vi "Convert Time to H_M_S.vi"(7 "Initial Scan Location":u32, 8 "error in":errorcluster, 10 "Tot. Timer Format":u16, 11 "Time Data String":string="Time Data String") -> (0 "error out":errorcluster, 1 "[sec]":dbl, 2 "[min]":dbl, 3 "[hr]":dbl, 5 "Offset Past Scan":u32)   [LabVIEW 2023]
doc: "Converts the Totalizer Timer data string into H:M:S doubles based on the time string format. A timer format of 2 is used if the Totalizer Timer is already outputting data in the H:M:S format.\n\nIf unsure of the format your Alicat uses, the output of the \"Read Measurement Format\" sub-VI will output the timer format for use with this sub-VI."
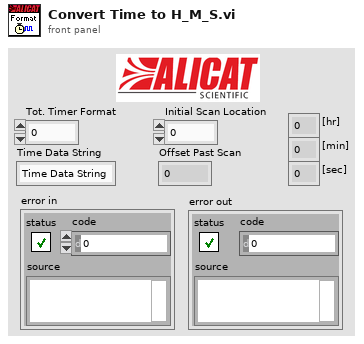
[diagram p1: front panel]
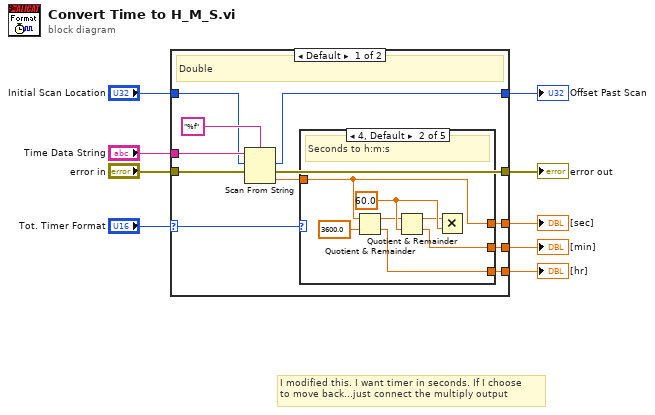
[diagram p0: block diagram]
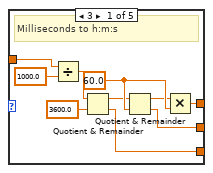
[diagram p2: hidden frame]
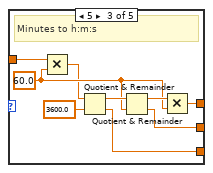
[diagram p3: hidden frame]
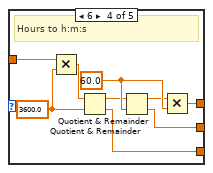
[diagram p4: hidden frame]
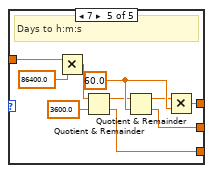
[diagram p5: hidden frame]
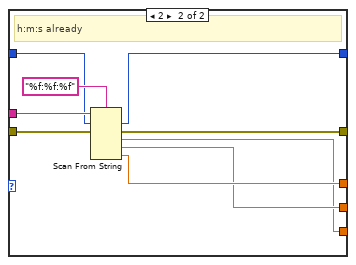
[diagram p6: hidden frame]
diagram:
  # "I modified this. I want timer in seconds. If I choose\nto move back...just connect the multiply output"
  n1 = case shown="Default" "Tot. Timer Format" {
    selector: "Tot. Timer Format" -> [w18 _]
    tunnel: "Time Data String" -> [w20 w74]
    tunnel: "error in" -> [w12 w72]
    tunnel: [w13 w71] -> w7
    tunnel: [w16 w70] -> w3
    tunnel: [w15 w69] -> w4
    tunnel: [w14 w68] -> w5
    tunnel: [w10 w67] -> w2
    tunnel: "Initial Scan Location" -> [w11 w66]
    frame Default {
      # "Double"
      n2 = Scan From String(format string="%f", input string=w20, initial scan location=w11, error in=w12) -> (offset past scan=w10:u32, error out=w13:errorcluster, output 1=w17:dbl)  [unwired: 1 in, 1 out]
      n3 = case shown="4, Default" w18 {
        tunnel: w17 -> [w29 w31 w40 w48 w64]
        tunnel: [w23 w31 w43 w50 w59] -> w16
        tunnel: [w22 w33 w42 w52 w58] -> w15
        tunnel: [w21 w32 w41 w51 w57] -> w14
        frame 3 {
          w28 = 60.0 ("y")
          # "Milliseconds to h:m:s"
          n4 = Divide(x=w29, y=1000.0) -> (x/y=w24:dbl)
          n5 = Quotient & Remainder(x=w24, y=3600.0) -> (x-y*floor(x/y)=w26:dbl, floor(x/y)=w21:dbl)
          n6 = Quotient & Remainder(x=w26, y=w28) -> (x-y*floor(x/y)=w27:dbl, floor(x/y)=w22:dbl)
          n7 = Multiply(x=w27, y=w28) -> (x*y=w23:dbl)
        }
        frame 4, Default {
          w37 = 60.0 ("y")
          # "Seconds to h:m:s"
          n8 = Quotient & Remainder(x=w31, y=3600.0) -> (x-y*floor(x/y)=w35:dbl, floor(x/y)=w32:dbl)
          n9 = Quotient & Remainder(x=w35, y=w37) -> (x-y*floor(x/y)=w36:dbl, floor(x/y)=w33:dbl)
          n10 = Multiply(x=w36, y=w37) -> ()  [unwired: 1 out]
        }
        frame 5 {
          w39 = 60.0 ("y")
          # "Minutes to h:m:s"
          n11 = Multiply(x=w40, y=w39) -> (x*y=w38:dbl)
          n12 = Quotient & Remainder(x=w38, y=3600.0) -> (x-y*floor(x/y)=w45:dbl, floor(x/y)=w41:dbl)
          n13 = Quotient & Remainder(x=w45, y=w39) -> (x-y*floor(x/y)=w46:dbl, floor(x/y)=w42:dbl)
          n14 = Multiply(x=w46, y=w39) -> (x*y=w43:dbl)
        }
        frame 6 {
          w55 = 60.0 ("y")
          w47 = 3600.0 ("y")
          # "Hours to h:m:s"
          n15 = Multiply(x=w48, y=w47) -> (x*y=w49:dbl)
          n16 = Quotient & Remainder(x=w49, y=w47) -> (x-y*floor(x/y)=w53:dbl, floor(x/y)=w51:dbl)
          n17 = Quotient & Remainder(x=w53, y=w55) -> (x-y*floor(x/y)=w54:dbl, floor(x/y)=w52:dbl)
          n18 = Multiply(x=w54, y=w55) -> (x*y=w50:dbl)
        }
        frame 7 {
          w63 = 60.0 ("y")
          # "Days to h:m:s"
          n19 = Multiply(x=w64, y=86400.0) -> (x*y=w56:dbl)
          n20 = Quotient & Remainder(x=w56, y=3600.0) -> (x-y*floor(x/y)=w61:dbl, floor(x/y)=w57:dbl)
          n21 = Quotient & Remainder(x=w61, y=w63) -> (x-y*floor(x/y)=w62:dbl, floor(x/y)=w58:dbl)
          n22 = Multiply(x=w62, y=w63) -> (x*y=w59:dbl)
        }
      }
    }
    frame 2 {
      # "h:m:s already"
      n23 = Scan From String(format string="%f:%f:%f", input string=w74, initial scan location=w66, error in=w72) -> (offset past scan=w67:u32, error out=w71:errorcluster, output 1=w68:dbl, output 2=w69:dbl, output 3=w70:dbl)  [unwired: 3 in, 1 out]
    }
  }
  "error out" <- w7
  "[hr]" <- w5
  "[min]" <- w4
  "[sec]" <- w3
  "Offset Past Scan" <- w2
